vi "Lab Panel V4.82.vi"() -> ()   [LabVIEW 2013] (continued)
            n287 = local read "jig cycle"() -> (w337:dbl)
            n288 = local read "on loops"() -> (w339:dbl)
            n289 = local read "off loops"() -> (w338:dbl)
            n290 = Add(x=w324, y=w323) -> (x+y=w322:dbl)
            n291 = Add(x=w339, y=w338) -> (x+y=w325:dbl)
            n292 = Greater Or Equal?(x=w337, y=w325) -> (x >= y?=w336:bool)
            n293 = case shown="True" w336 {
              tunnel: w335 -> [_ w372]
              tunnel: w334 -> [_ w371]
              tunnel: w333 -> [_ w370]
              tunnel: w332 -> [_ w369]
              tunnel: w331 -> [_ w368]
              tunnel: w330 -> [_ w367]
              tunnel: w329 -> [_ w366]
              tunnel: w328 -> [_ w365]
              tunnel: w327 -> [_ w364]
              tunnel: w326 -> [_ w363]
              tunnel: w322 -> [_ w362]
              frame False {
              }
              frame True {
                # "increment cycle value and convert cycles to minutes for temp rise"
                n294 = local read "JIG RELAY CYCLES"() -> (w361:T10)
                n295 = Unbundle By Name(w361) -> ("LAB01-1"=w359:dbl, "LAB01-2"=w357:dbl, "LAB02-1"=w355:dbl, "LAB02-2"=w353:dbl, "LAB03-1"=w351:dbl, "LAB03-2"=w349:dbl, "LAB04-1"=w347:dbl, "LAB04-2"=w345:dbl, "LAB05-1"=w343:dbl, "LAB05-2"=w341:dbl)
                n296 = stacked-sequence {
                  tunnel: w372 -> [w384 _ _ _ _ _ _ _ _ _]
                  tunnel: w371 -> [_ w401 _ _ _ _ _ _ _ _]
                  tunnel: w370 -> [_ _ w418 _ _ _ _ _ _ _]
                  tunnel: w369 -> [_ _ _ w435 _ _ _ _ _ _]
                  tunnel: w368 -> [_ _ _ _ w452 _ _ _ _ _]
                  tunnel: w367 -> [_ _ _ _ _ w469 _ _ _ _]
                  tunnel: w366 -> [_ _ _ _ _ _ w486 _ _ _]
                  tunnel: w365 -> [_ _ _ _ _ _ _ w503 _ _]
                  tunnel: w364 -> [_ _ _ _ _ _ _ _ w520 _]
                  tunnel: w363 -> [_ _ _ _ _ _ _ _ _ w537]
                  tunnel: w362 -> [w381 w398 w415 w432 w449 w466 w483 w500 w517 w534]
                  tunnel: w359 -> [w375 _ _ _ _ _ _ _ _ _]
                  tunnel: [w374 _ _ _ _ _ _ _ _ _] -> w358
                  tunnel: w357 -> [_ w392 _ _ _ _ _ _ _ _]
                  tunnel: [_ w391 _ _ _ _ _ _ _ _] -> w356
                  tunnel: w355 -> [_ _ w409 _ _ _ _ _ _ _]
                  tunnel: [_ _ w408 _ _ _ _ _ _ _] -> w354
                  tunnel: w353 -> [_ _ _ w426 _ _ _ _ _ _]
                  tunnel: [_ _ _ w425 _ _ _ _ _ _] -> w352
                  tunnel: w351 -> [_ _ _ _ w443 _ _ _ _ _]
                  tunnel: [_ _ _ _ w442 _ _ _ _ _] -> w350
                  tunnel: w349 -> [_ _ _ _ _ w460 _ _ _ _]
                  tunnel: [_ _ _ _ _ w459 _ _ _ _] -> w348
                  tunnel: w347 -> [_ _ _ _ _ _ w477 _ _ _]
                  tunnel: [_ _ _ _ _ _ w476 _ _ _] -> w346
                  tunnel: w345 -> [_ _ _ _ _ _ _ w494 _ _]
                  tunnel: [_ _ _ _ _ _ _ w493 _ _] -> w344
                  tunnel: w343 -> [_ _ _ _ _ _ _ _ w511 _]
                  tunnel: [_ _ _ _ _ _ _ _ w510 _] -> w342
                  tunnel: w341 -> [_ _ _ _ _ _ _ _ _ w528]
                  tunnel: [_ _ _ _ _ _ _ _ _ w527] -> w340
                  frame #0 {
                    n297 = local read "DISP LAB01-1"() -> (w379:T4)
                    n298 = Unbundle(w379) -> ("CYCLE"=w380:dbl)  [unwired: 2 out]
                    n299 = case shown="True" w384 {
                      tunnel: w380 -> [w386 w390]
                      tunnel: [w386 w389] -> w378
                      tunnel: w375 -> [w385 w388]
                      tunnel: [w385 w387] -> w374
                      frame False {
                      }
                      frame True {
                        n300 = Increment(x=w388) -> (x+1=w387:dbl)
                        n301 = Increment(x=w390) -> (x+1=w389:dbl)
                      }
                    }
                    n302 = Multiply(x=w378, y=w381) -> (x*y=w382:dbl)
                    n303 = Divide(x=w382, y=60.0) -> (x/y=w377:dbl)
                    n304 = Bundle(cluster=w379, "CYCLE"=w378, "MINS"=w377) -> (w376:T4)  [unwired: 1 in]
                    n305 = local write "DISP LAB01-1"(w376) -> ()
                  }
                  frame #1 {
                    n306 = local read "DISP LAB01-2"() -> (w396:T4)
                    n307 = Unbundle(w396) -> ("CYCLE"=w397:dbl)  [unwired: 2 out]
                    n308 = case shown="True" w401 {
                      tunnel: w397 -> [w403 w407]
                      tunnel: [w403 w406] -> w394
                      tunnel: w392 -> [w402 w405]
                      tunnel: [w402 w404] -> w391
                      frame False {
                      }
                      frame True {
                        n309 = Increment(x=w405) -> (x+1=w404:dbl)
                        n310 = Increment(x=w407) -> (x+1=w406:dbl)
                      }
                    }
                    n311 = Multiply(x=w394, y=w398) -> (x*y=w399:dbl)
                    n312 = Divide(x=w399, y=60.0) -> (x/y=w393:dbl)
                    n313 = Bundle(cluster=w396, "CYCLE"=w394, "MINS"=w393) -> (w395:T4)  [unwired: 1 in]
                    n314 = local write "DISP LAB01-2"(w395) -> ()
                  }
                  frame #2 {
                    n315 = local read "DISP LAB02-1"() -> (w413:T4)
                    n316 = Unbundle(w413) -> ("CYCLE"=w414:dbl)  [unwired: 2 out]
                    n317 = case shown="True" w418 {
                      tunnel: [w420 w424] -> w411
                      tunnel: w414 -> [w420 w423]
                      tunnel: w409 -> [w419 w422]
                      tunnel: [w419 w421] -> w408
                      frame False {
                      }
                      frame True {
                        n318 = Increment(x=w422) -> (x+1=w421:dbl)
                        n319 = Increment(x=w423) -> (x+1=w424:dbl)
                      }
                    }
                    n320 = Multiply(x=w411, y=w415) -> (x*y=w416:dbl)
                    n321 = Divide(x=w416, y=60.0) -> (x/y=w410:dbl)
                    n322 = Bundle(cluster=w413, "CYCLE"=w411, "MINS"=w410) -> (w412:T4)  [unwired: 1 in]
                    n323 = local write "DISP LAB02-1"(w412) -> ()
                  }
                  frame #3 {
                    n324 = local read "DISP LAB02-2"() -> (w430:T4)
                    n325 = Unbundle(w430) -> ("CYCLE"=w431:dbl)  [unwired: 2 out]
                    n326 = case shown="True" w435 {
                      tunnel: [w437 w441] -> w429
                      tunnel: w431 -> [w437 w440]
                      tunnel: w426 -> [w436 w439]
                      tunnel: [w436 w438] -> w425
                      frame False {
                      }
                      frame True {
                        n327 = Increment(x=w439) -> (x+1=w438:dbl)
                        n328 = Increment(x=w440) -> (x+1=w441:dbl)
                      }
                    }
                    n329 = Multiply(x=w429, y=w432) -> (x*y=w433:dbl)
                    n330 = Divide(x=w433, y=60.0) -> (x/y=w428:dbl)
                    n331 = Bundle(cluster=w430, "CYCLE"=w429, "MINS"=w428) -> (w427:T4)  [unwired: 1 in]
                    n332 = local write "DISP LAB02-2"(w427) -> ()
                  }
                  frame #4 {
                    n333 = local read "DISP LAB03-1"() -> (w447:T4)
                    n334 = Unbundle(w447) -> ("CYCLE"=w448:dbl)  [unwired: 2 out]
                    n335 = case shown="True" w452 {
                      tunnel: [w454 w458] -> w444
                      tunnel: w448 -> [w454 w457]
                      tunnel: w443 -> [w453 w456]
                      tunnel: [w453 w455] -> w442
                      frame False {
                      }
                      frame True {
                        n336 = Increment(x=w456) -> (x+1=w455:dbl)
                        n337 = Increment(x=w457) -> (x+1=w458:dbl)
                      }
                    }
                    n338 = Multiply(x=w444, y=w449) -> (x*y=w450:dbl)
                    n339 = Divide(x=w450, y=60.0) -> (x/y=w445:dbl)
                    n340 = Bundle(cluster=w447, "CYCLE"=w444, "MINS"=w445) -> (w446:T4)  [unwired: 1 in]
                    n341 = local write "DISP LAB03-1"(w446) -> ()
                  }
                  frame #5 {
                    n342 = local read "DISP LAB03-2"() -> (w464:T4)
                    n343 = Unbundle(w464) -> ("CYCLE"=w465:dbl)  [unwired: 2 out]
                    n344 = case shown="True" w469 {
                      tunnel: [w471 w475] -> w463
                      tunnel: w465 -> [w471 w474]
                      tunnel: w460 -> [w470 w473]
                      tunnel: [w470 w472] -> w459
                      frame False {
                      }
                      frame True {
                        n345 = Increment(x=w473) -> (x+1=w472:dbl)
                        n346 = Increment(x=w474) -> (x+1=w475:dbl)
                      }
                    }
                    n347 = Multiply(x=w463, y=w466) -> (x*y=w467:dbl)
                    n348 = Divide(x=w467, y=60.0) -> (x/y=w462:dbl)
                    n349 = Bundle(cluster=w464, "CYCLE"=w463, "MINS"=w462) -> (w461:T4)  [unwired: 1 in]
                    n350 = local write "DISP LAB03-2"(w461) -> ()
                  }
                  frame #6 {
                    n351 = local read "DISP LAB04-1"() -> (w481:T4)
                    n352 = Unbundle(w481) -> ("CYCLE"=w482:dbl)  [unwired: 2 out]
                    n353 = case shown="True" w486 {
                      tunnel: [w488 w492] -> w479
                      tunnel: w482 -> [w488 w491]
                      tunnel: w477 -> [w487 w490]
                      tunnel: [w487 w489] -> w476
                      frame False {
                      }
                      frame True {
                        n354 = Increment(x=w490) -> (x+1=w489:dbl)
                        n355 = Increment(x=w491) -> (x+1=w492:dbl)
                      }
                    }
                    n356 = Multiply(x=w479, y=w483) -> (x*y=w484:dbl)
                    n357 = Divide(x=w484, y=60.0) -> (x/y=w478:dbl)
                    n358 = Bundle(cluster=w481, "CYCLE"=w479, "MINS"=w478) -> (w480:T4)  [unwired: 1 in]
                    n359 = local write "DISP LAB04-1"(w480) -> ()
                  }
                  frame #7 {
                    n360 = local read "DISP LAB04-2"() -> (w498:T4)
                    n361 = Unbundle(w498) -> ("CYCLE"=w499:dbl)  [unwired: 2 out]
                    n362 = case shown="True" w503 {
                      tunnel: [w505 w509] -> w496
                      tunnel: w499 -> [w505 w508]
                      tunnel: w494 -> [w504 w507]
                      tunnel: [w504 w506] -> w493
                      frame False {
                      }
                      frame True {
                        n363 = Increment(x=w507) -> (x+1=w506:dbl)
                        n364 = Increment(x=w508) -> (x+1=w509:dbl)
                      }
                    }
                    n365 = Multiply(x=w496, y=w500) -> (x*y=w502:dbl)
                    n366 = Divide(x=w502, y=60.0) -> (x/y=w495:dbl)
                    n367 = Bundle(cluster=w498, "CYCLE"=w496, "MINS"=w495) -> (w497:T4)  [unwired: 1 in]
                    n368 = local write "DISP LAB04-2"(w497) -> ()
                  }
                  frame #8 {
                    n369 = local read "DISP LAB05-1"() -> (w515:T4)
                    n370 = Unbundle(w515) -> ("CYCLE"=w516:dbl)  [unwired: 2 out]
                    n371 = case shown="True" w520 {
                      tunnel: [w522 w526] -> w513
                      tunnel: w516 -> [w522 w525]
                      tunnel: w511 -> [w521 w524]
                      tunnel: [w521 w523] -> w510
                      frame False {
                      }
                      frame True {
                        n372 = Increment(x=w524) -> (x+1=w523:dbl)
                        n373 = Increment(x=w525) -> (x+1=w526:dbl)
                      }
                    }
                    n374 = Multiply(x=w513, y=w517) -> (x*y=w518:dbl)
                    n375 = Divide(x=w518, y=60.0) -> (x/y=w512:dbl)
                    n376 = Bundle(cluster=w515, "CYCLE"=w513, "MINS"=w512) -> (w514:T4)  [unwired: 1 in]
                    n377 = local write "DISP LAB05-1"(w514) -> ()
                  }
                  frame #9 {
                    n378 = local read "DISP LAB05-2"() -> (w533:T4)
                    n379 = Unbundle(w533) -> ("CYCLE"=w532:dbl)  [unwired: 2 out]
                    n380 = case shown="True" w537 {
                      tunnel: [w539 w543] -> w531
                      tunnel: w532 -> [w539 w542]
                      tunnel: w528 -> [w538 w541]
                      tunnel: [w538 w540] -> w527
                      frame False {
                      }
                      frame True {
                        n381 = Increment(x=w541) -> (x+1=w540:dbl)
                        n382 = Increment(x=w542) -> (x+1=w543:dbl)
                      }
                    }
                    n383 = Multiply(x=w531, y=w534) -> (x*y=w535:dbl)
                    n384 = Divide(x=w535, y=60.0) -> (x/y=w530:dbl)
                    n385 = Bundle(cluster=w533, "CYCLE"=w531, "MINS"=w530) -> (w529:T4)  [unwired: 1 in]
                    n386 = local write "DISP LAB05-2"(w529) -> ()
                  }
                }
                n387 = local write "jig cycle"(0) -> ()
                n388 = Bundle By Name(cluster=w361, "LAB01-1"=w358, "LAB01-2"=w356, "LAB02-1"=w354, "LAB02-2"=w352, "LAB03-1"=w350, "LAB03-2"=w348, "LAB04-1"=w346, "LAB04-2"=w344, "LAB05-1"=w342, "LAB05-2"=w340) -> (w360:T10)
                n389 = local write "JIG RELAY CYCLES"(w360) -> ()
              }
            }
          }
          frame #3 {
            # "START & STOP test RUN switch change, start test if true and stop test if false"
            n390 = Get Date/Time In Seconds() -> (seconds since 1Jan1904=w551:timestamp)
            n391 = local read "C drive data root dir"() -> (w544:path)
            n392 = Format Date/Time String(time format string (%c)="%b\\%a%d", seconds (now)=w551) -> (date/time string=w575:string)  [unwired: 1 in]
            n393 = Format Date/Time String(time format string (%c)="%H%M", seconds (now)=w551) -> (date/time string=w573:string)  [unwired: 1 in]
            n394 = Format Date/Time String(time format string (%c)="LabPanel%Y", seconds (now)=w551) -> (date/time string=w550:string)  [unwired: 1 in]
            n395 = Path To String(path=w544) -> (string=w547:string)
            n396 = global write "Global 1.vi" "C drive root path"(w544) -> ()
            n397 = Concatenate Strings(w547, "\\") -> (w545:string)
            n398 = event shown="[5] \"RUN LAB03-1\": Value Change" {
              selector: _ -> [_ _ _ _ _ _ _ _ _ _ _]
              dyn-events: _ -> [_ _ _ _ _ _ _ _ _ _ _]
              timeout: 10 -> [_ _ _ _ _ _ _ _ _ _ _]
              tunnel: w545 -> [_ w583 w675 w767 w859 w951 w1043 w1135 w1227 w1319 w1411]
              tunnel: w575 -> [_ w582 w674 w766 w858 w950 w1042 w1134 w1226 w1318 w1410]
              tunnel: w573 -> [_ w580 w673 w765 w857 w949 w1041 w1133 w1225 w1317 w1409]
              tunnel: w571 -> [_ w581 _ _ _ _ _ _ _ _ _]
              tunnel: w572 -> [_ _ _ _ _ _ _ _ _ _ _]
              tunnel: w570 -> [_ _ _ _ _ _ _ _ _ _ _]
              tunnel: w569 -> [_ _ w672 _ _ _ _ _ _ _ _]
              tunnel: w568 -> [_ _ _ _ _ _ _ _ _ _ _]
              tunnel: w567 -> [_ _ _ w764 _ _ _ _ _ _ _]
              tunnel: w566 -> [_ _ _ _ _ _ _ _ _ _ _]
              tunnel: w565 -> [_ _ _ _ w856 _ _ _ _ _ _]
              tunnel: w564 -> [_ _ _ _ _ _ _ _ _ _ _]
              tunnel: w563 -> [_ _ _ _ _ w948 _ _ _ _ _]
              tunnel: w562 -> [_ _ _ _ _ _ _ _ _ _ _]
              tunnel: w561 -> [_ _ _ _ _ _ w1040 _ _ _ _]
              tunnel: w560 -> [_ _ _ _ _ _ _ _ _ _ _]
              tunnel: w559 -> [_ _ _ _ _ _ _ w1132 _ _ _]
              tunnel: w558 -> [_ _ _ _ _ _ _ _ _ _ _]
              tunnel: w557 -> [_ _ _ _ _ _ _ _ w1224 _ _]
              tunnel: w556 -> [_ _ _ _ _ _ _ _ _ _ _]
              tunnel: w555 -> [_ _ _ _ _ _ _ _ _ w1316 _]
              tunnel: w554 -> [_ _ _ _ _ _ _ _ _ _ _]
              tunnel: w553 -> [_ _ _ _ _ _ _ _ _ _ w1408]
              tunnel: w550 -> [_ w579 w671 w763 w855 w947 w1039 w1131 w1223 w1315 w1407]
              tunnel: [_ w578 w670 w762 w854 w946 w1038 w1130 w1222 w1314 w1406] -> w548
              event Timeout {
                n399 = event-data() -> ()  [unwired: 1 in, 3 out]
              }
              event "RUN LAB01-1": Value Change {
                n400 = event-data() -> ("NewVal"=w577:bool)  [unwired: 1 in, 5 out]
                n401 = local write "run lab01-1"(w577) -> ()
                n402 = case shown="True" w577 {
                  tunnel: w583 -> [_ w616]
                  tunnel: w582 -> [_ w615]
                  tunnel: w581 -> [w585 w614]
                  tunnel: w580 -> [_ w613]
                  tunnel: w579 -> [_ w612]
                  tunnel: [w584 w611] -> w578
                  frame False {
                    # "stop test"
                    n403 = stacked-sequence {
                      tunnel: w585 -> [_ w597 _ _]
                      tunnel: [_ w589 _ _] -> w584
                      frame #0 {
                        n404 = local read "DISP LAB01-1"() -> (w588:T4)
                        n405 = Bundle(cluster=w588, "STATUS"="STOP") -> (w586:T4)  [unwired: 2 in]
                        n406 = local write "DISP LAB01-1"(w586) -> ()
                      }
                      frame #1 {
                        n407 = local read "DISP LAB01-1"() -> (w596:T4)
                        n408 = Unbundle(w596) -> ("CYCLE"=w594:dbl, "MINS"=w595:dbl)  [unwired: 1 out]
                        n409 = case shown="\"CYCLE TEST\"" w597 {
                          tunnel: w595 -> [_ _ w604]
                          tunnel: w594 -> [w602 w603 _]
                          tunnel: [w602 w603 w604] -> w593
                          frame "CHART TEST", Default {
                          }
                          frame "CYCLE TEST" {
                          }
                          frame "T-RISE TEST" {
                          }
                        }
                        n410 = local read "TDMS LAB01-1"() -> (w601:refnum<k34>)
                        n411 = Build Array("STOPPED") -> (w598:string[])
                        n412 = Build Array(w593) -> (w592:dbl[])
                        n413 = TDMS Write(0:w601, 5:"TEST RESULT", 7:w598, 9:w592) -> (4:w590:refnum<k34>, 15:w591:errorcluster)  [unwired: 2 in, 2 out]
                        n414 = TDMS Close(8:w591, 11:w590) -> (0:w589:errorcluster)  [unwired: 1 out]
                      }
                      frame #2 {
                        n415 = stacked-sequence {
                          tunnel: "LAB01-1" -> [w607 w609]
                          frame #0 {
                            n416 = call "sub vi - defrag tdms v1.vi"("panel id"=w607) -> ("error out"=w606:errorcluster)  [unwired: 10 in]
                            n417 = local write "data file error"(w606) -> ()
                          }
                          frame #1 {
                            n418 = call "Save data file to network drive v1.vi"("panel id"=w609) -> ("network file save error"=w608:errorcluster)  [unwired: 9 in, 1 out]
                            n419 = local write "RESULT LAB01-1"(FALSE) -> ()
                            n420 = local write "data file error"(w608) -> ()
                          }
                        }
                      }
                      frame #3 {
                      }
                    }
                  }
                  frame True {
                    # "start new test and create test file"
                    n421 = stacked-sequence {
                      seq-local: [w617 _ _ _ _] -> [_ w638 _ _ _]
                      tunnel: w616 -> [w622 _ _ _ _]
                      tunnel: w615 -> [w618 _ _ _ _]
                      tunnel: w614 -> [w632 _ _ _ _]
                      tunnel: w613 -> [w625 _ _ _ _]
                      tunnel: w612 -> [w620 _ _ _ _]
                      tunnel: [_ w639 _ _ _] -> w611
                      frame #0 {
                        w619 = "\\"
                        n422 = case shown="\"CHART TEST\", Default" w632 {
                          tunnel: ["L01-1-CHART TEST-" "L01-1-CYCLE TEST-" "L01-1-T-RISE TEST-"] -> w628
                          frame "CHART TEST", Default {
                          }
                          frame "CYCLE TEST" {
                          }
                          frame "T-RISE TEST" {
                          }
                        }
                        n423 = local read "SET LAB01-1"() -> (w627:T5)
                        n424 = Unbundle(w627) -> ("DESCRIPTION"=w626:string)  [unwired: 4 out]
                        n425 = Concatenate Strings(w622, "\\", w620, w619, w618, w619) -> (w629:string)
                        n426 = String To Path(string=w629) -> (path=w631:path)
                        n427 = Concatenate Strings(w629, w628, w626, "-", w625, ".tdms") -> (w617:string)
                        n428 = Create Folder(path (use dialog)=w631) -> (error out=w630:errorcluster)  [unwired: 2 in, 2 out]
                        n429 = call <vilib>:"Clear Errors.vi"("error in (no error)"=w630) -> ()  [unwired: 6 in, 1 out]
                        n430 = global write "Global 1.vi" "LAB01-1 FILE"(w617) -> ()
                      }
                      frame #1 {
                        n431 = String To Path(string=w638) -> (path=w636:path)
                        n432 = TDMS Open(5:FALSE, 6:FALSE, 10:T19."create or replace" ("operation (0:open)"), 11:w636) -> (0:w639:errorcluster, 3:→"TDMS LAB01-1":refnum<k34>)  [unwired: 3 in]
                      }
                      frame #2 {
                        n433 = local read "TDMS LAB01-1"() -> (w659:refnum<k34>)
                        n434 = local read "SET LAB01-1"() -> (w648:T5)
                        n435 = Build Array("Testers Name", "Description", "Set Test Cycles", "T-Rise minutes", "T-Rise Deg C") -> (w649:string[])
                        n436 = Unbundle(w648) -> ("NAME"=w647:string, "DESCRIPTION"=w646:string, "CYCLES"=w645:dbl, "T-RISE mins"=w644:dbl, "T-RISE deg C"=w643:dbl)
                        n437 = Number To Decimal String(number=w645) -> (decimal integer string=w658:string)  [unwired: 1 in]
                        n438 = Number To Decimal String(number=w644) -> (decimal integer string=w657:string)  [unwired: 1 in]
                        n439 = Number To Decimal String(number=w643) -> (decimal integer string=w656:string)  [unwired: 1 in]
                        n440 = Build Array(w647, w646, w658, w657, w656) -> (w655:string[])
                        n441 = TDMS Set Properties(5:w655, 7:w649, 11:w659) -> ()  [unwired: 3 in, 4 out]
                      }
                      frame #3 {
                        w660 = 0.0
                        n442 = local read "DISP LAB01-1"() -> (w663:T4)
                        n443 = Bundle(cluster=w663, "CYCLE"=w660, "MINS"=w660, "STATUS"="RUN") -> (w662:T4)
                        n444 = local write "DISP LAB01-1"(w662) -> ()
                      }
                      frame #4 {
                        n445 = local read "SIG LAB01-1"() -> (w666:T2)
                        n446 = local read "TEMP START LAB01-1"() -> (w668:cluster{"TL":dbl, "TN":dbl})
                        n447 = Unbundle(w666) -> ("Tmp Live"=w665:dbl, "Tmp Neut"=w664:dbl)  [unwired: 3 out]
                        n448 = Bundle(cluster=w668, "TL"=w665, "TN"=w664) -> (w667:cluster{"TL":dbl, "TN":dbl})
                        n449 = local write "TEMP START LAB01-1"(w667) -> ()
                      }
                    }
                  }
                }
              }
              event "RUN LAB01-2": Value Change {
                n450 = event-data() -> ("NewVal"=w669:bool)  [unwired: 1 in, 5 out]
                n451 = local write "run lab01-2"(w669) -> ()
                n452 = case shown="True" w669 {
                  tunnel: w675 -> [_ w708]
                  tunnel: w674 -> [_ w707]
                  tunnel: w672 -> [w677 w706]
                  tunnel: w673 -> [_ w705]
                  tunnel: w671 -> [_ w704]
                  tunnel: [w676 w703] -> w670
                  frame False {
                    # "stop test"
                    n453 = stacked-sequence {
                      tunnel: w677 -> [w686 _]
                      tunnel: [w678 _] -> w676
                      frame #0 {
                        n454 = local read "DISP LAB01-2"() -> (w685:T4)
                        n455 = Unbundle(w685) -> ("CYCLE"=w683:dbl, "MINS"=w684:dbl)  [unwired: 1 out]
                        n456 = case shown="\"CHART TEST\", Default" w686 {
                          tunnel: w684 -> [_ _ w693]
                          tunnel: w683 -> [w691 w692 _]
                          tunnel: [w691 w692 w693] -> w682
                          frame "CHART TEST", Default {
                          }
                          frame "CYCLE TEST" {
                          }
                          frame "T-RISE TEST" {
                          }
                        }
                        n457 = local read "TDMS LAB01-2"() -> (w690:refnum<k34>)
                        n458 = Build Array("STOPPED") -> (w687:string[])
                        n459 = Build Array(w682) -> (w681:dbl[])
                        n460 = TDMS Write(0:w690, 5:"TEST RESULT", 7:w687, 9:w681) -> (4:w679:refnum<k34>, 15:w680:errorcluster)  [unwired: 2 in, 2 out]
                        n461 = TDMS Close(8:w680, 11:w679) -> (0:w678:errorcluster)  [unwired: 1 out]
                      }
                      frame #1 {
                        n462 = local read "DISP LAB01-2"() -> (w697:T4)
                        n463 = stacked-sequence {
                          tunnel: "LAB01-2" -> [w699 w701]
                          frame #0 {
                            n464 = call "sub vi - defrag tdms v1.vi"("panel id"=w699) -> ("error out"=w698:errorcluster)  [unwired: 10 in]
                            n465 = local write "data file error"(w698) -> ()
                          }
                          frame #1 {
                            n466 = call "Save data file to network drive v1.vi"("panel id"=w701) -> ("network file save error"=w700:errorcluster)  [unwired: 9 in, 1 out]
                            n467 = local write "RESULT LAB01-2"(FALSE) -> ()
                            n468 = local write "data file error"(w700) -> ()
                          }
                        }
                        n469 = Bundle(cluster=w697, "STATUS"="STOP") -> (w695:T4)  [unwired: 2 in]
                        n470 = local write "DISP LAB01-2"(w695) -> ()
                      }
                    }
                  }
                  frame True {
                    # "start new test and create test file"
                    n471 = stacked-sequence {
                      seq-local: [w709 _ _ _ _] -> [_ w734 _ _ _]
                      tunnel: w708 -> [w714 _ _ _ _]
                      tunnel: w707 -> [w711 _ _ _ _]
                      tunnel: w706 -> [w724 _ _ _ _]
                      tunnel: w705 -> [w717 _ _ _ _]
                      tunnel: w704 -> [w712 _ _ _ _]
                      tunnel: [_ w728 _ _ _] -> w703
                      frame #0 {
                        w710 = "\\"
                        n472 = local read "SET LAB01-2"() -> (w719:T5)
                        n473 = case shown="\"CYCLE TEST\"" w724 {
                          tunnel: ["L01-2-CHART TEST-" "L01-2-CYCLE TEST-" "L01-2-T-RISE TEST-"] -> w720
                          frame "CHART TEST", Default {
                          }
                          frame "CYCLE TEST" {
                          }
                          frame "T-RISE TEST" {
                          }
                        }
                        n474 = Unbundle(w719) -> ("DESCRIPTION"=w718:string)  [unwired: 4 out]
                        n475 = Concatenate Strings(w714, "\\", w712, w710, w711, w710) -> (w721:string)
                        n476 = String To Path(string=w721) -> (path=w723:path)
                        n477 = Concatenate Strings(w721, w720, w718, "-", w717, ".tdms") -> (w709:string)
                        n478 = Create Folder(path (use dialog)=w723) -> (error out=w722:errorcluster)  [unwired: 2 in, 2 out]
                        n479 = global write "Global 1.vi" "LAB01-2 FILE"(w709) -> ()
                        n480 = call <vilib>:"Clear Errors.vi"("error in (no error)"=w722) -> ()  [unwired: 6 in, 1 out]
                      }
                      frame #1 {
                        n481 = String To Path(string=w734) -> (path=w729:path)
                        n482 = TDMS Open(5:FALSE, 6:FALSE, 10:T19."create or replace" ("operation (0:open)"), 11:w729) -> (0:w728:errorcluster, 3:→"TDMS LAB01-2":refnum<k34>)  [unwired: 3 in]
                      }
                      frame #2 {
                        n483 = local read "SET LAB01-2"() -> (w740:T5)
                        n484 = local read "TDMS LAB01-2"() -> (w751:refnum<k34>)
                        n485 = Build Array("Testers Name", "Description", "Set Test Cycles", "T-Rise minutes", "T-Rise Deg C") -> (w741:string[])
                        n486 = Unbundle(w740) -> ("NAME"=w739:string, "DESCRIPTION"=w738:string, "CYCLES"=w737:dbl, "T-RISE mins"=w736:dbl, "T-RISE deg C"=w735:dbl)
                        n487 = Number To Decimal String(number=w737) -> (decimal integer string=w750:string)  [unwired: 1 in]
                        n488 = Number To Decimal String(number=w736) -> (decimal integer string=w749:string)  [unwired: 1 in]
                        n489 = Number To Decimal String(number=w735) -> (decimal integer string=w748:string)  [unwired: 1 in]
                        n490 = Build Array(w739, w738, w750, w749, w748) -> (w747:string[])
                        n491 = TDMS Set Properties(5:w747, 7:w741, 11:w751) -> ()  [unwired: 3 in, 4 out]
                      }
                      frame #3 {
                        w753 = 0.0
                        n492 = local read "DISP LAB01-2"() -> (w755:T4)
                        n493 = Bundle(cluster=w755, "CYCLE"=w753, "MINS"=w753, "STATUS"="RUN") -> (w754:T4)
                        n494 = local write "DISP LAB01-2"(w754) -> ()
                      }
                      frame #4 {
                        n495 = local read "SIG LAB01-2"() -> (w758:T2)
                        n496 = local read "TEMP START LAB01-2"() -> (w760:cluster{"TL":dbl, "TN":dbl})
                        n497 = Unbundle(w758) -> ("Tmp Live"=w757:dbl, "Tmp Neut"=w756:dbl)  [unwired: 3 out]
                        n498 = Bundle(cluster=w760, "TL"=w757, "TN"=w756) -> (w759:cluster{"TL":dbl, "TN":dbl})
                        n499 = local write "TEMP START LAB01-2"(w759) -> ()
                      }
                    }
                  }
                }
              }
              event "RUN LAB02-1": Value Change {
                n500 = event-data() -> ("NewVal"=w761:bool)  [unwired: 1 in, 5 out]
                n501 = local write "run lab02-1"(w761) -> ()
                n502 = case shown="True" w761 {
                  tunnel: w767 -> [_ w800]
                  tunnel: w766 -> [_ w799]
                  tunnel: w764 -> [w769 w798]
                  tunnel: w765 -> [_ w797]
                  tunnel: w763 -> [_ w796]
                  tunnel: [w768 w795] -> w762
                  frame False {
                    # "stop test"
                    n503 = stacked-sequence {
                      tunnel: w769 -> [w778 _]
                      tunnel: [w770 _] -> w768
                      frame #0 {
                        n504 = local read "DISP LAB02-1"() -> (w777:T4)
                        n505 = Unbundle(w777) -> ("CYCLE"=w775:dbl, "MINS"=w776:dbl)  [unwired: 1 out]
                        n506 = case shown="\"CYCLE TEST\"" w778 {
                          tunnel: w776 -> [_ _ w785]
                          tunnel: w775 -> [w783 w784 _]
                          tunnel: [w783 w784 w785] -> w774
                          frame "CHART TEST", Default {
                          }
                          frame "CYCLE TEST" {
                          }
                          frame "T-RISE TEST" {
                          }
                        }
                        n507 = local read "TDMS LAB02-1"() -> (w782:refnum<k34>)
                        n508 = Build Array("STOPPED") -> (w779:string[])
                        n509 = Build Array(w774) -> (w773:dbl[])
                        n510 = TDMS Write(0:w782, 5:"TEST RESULT", 7:w779, 9:w773) -> (4:w771:refnum<k34>, 15:w772:errorcluster)  [unwired: 2 in, 2 out]
                        n511 = TDMS Close(8:w772, 11:w771) -> (0:w770:errorcluster)  [unwired: 1 out]
                      }
                      frame #1 {
                        n512 = local read "DISP LAB02-1"() -> (w789:T4)
                        n513 = stacked-sequence {
                          tunnel: "LAB02-1" -> [w791 w793]
                          frame #0 {
                            n514 = call "sub vi - defrag tdms v1.vi"("panel id"=w791) -> ("error out"=w790:errorcluster)  [unwired: 10 in]
                            n515 = local write "data file error"(w790) -> ()
                          }
                          frame #1 {
                            n516 = local write "RESULT LAB02-1"(FALSE) -> ()
                            n517 = call "Save data file to network drive v1.vi"("panel id"=w793) -> ("network file save error"=w792:errorcluster)  [unwired: 9 in, 1 out]
                            n518 = local write "data file error"(w792) -> ()
                          }
                        }
                        n519 = Bundle(cluster=w789, "STATUS"="STOP") -> (w787:T4)  [unwired: 2 in]
                        n520 = local write "DISP LAB02-1"(w787) -> ()
                      }
                    }
                  }
                  frame True {
                    # "start new test and create test file"
                    n521 = stacked-sequence {
                      seq-local: [w801 _ _ _ _] -> [_ w826 _ _ _]
                      tunnel: w800 -> [w806 _ _ _ _]
                      tunnel: w799 -> [w803 _ _ _ _]
                      tunnel: w798 -> [w816 _ _ _ _]
                      tunnel: w797 -> [w809 _ _ _ _]
                      tunnel: w796 -> [w804 _ _ _ _]
                      tunnel: [_ w820 _ _ _] -> w795
                      frame #0 {
                        w802 = "\\"
                        n522 = local read "SET LAB02-1"() -> (w811:T5)
                        n523 = case shown="\"CYCLE TEST\"" w816 {
                          tunnel: ["L02-1-CHART TEST-" "L02-1-CYCLE TEST-" "L02-1-T-RISE TEST-"] -> w812
                          frame "CHART TEST", Default {
                          }
                          frame "CYCLE TEST" {
                          }
                          frame "T-RISE TEST" {
                          }
                        }
                        n524 = Unbundle(w811) -> ("DESCRIPTION"=w810:string)  [unwired: 4 out]
                        n525 = Concatenate Strings(w806, "\\", w804, w802, w803, w802) -> (w813:string)
                        n526 = String To Path(string=w813) -> (path=w815:path)
                        n527 = Concatenate Strings(w813, w812, w810, "-", w809, ".tdms") -> (w801:string)
                        n528 = Create Folder(path (use dialog)=w815) -> (error out=w814:errorcluster)  [unwired: 2 in, 2 out]
                        n529 = global write "Global 1.vi" "LAB02-1 FILE"(w801) -> ()
                        n530 = call <vilib>:"Clear Errors.vi"("error in (no error)"=w814) -> ()  [unwired: 6 in, 1 out]
                      }
                      frame #1 {
                        n531 = String To Path(string=w826) -> (path=w821:path)
                        n532 = TDMS Open(5:FALSE, 6:FALSE, 10:T19."create or replace" ("operation (0:open)"), 11:w821) -> (0:w820:errorcluster, 3:→"TDMS LAB02-1":refnum<k34>)  [unwired: 3 in]
                      }
                      frame #2 {
                        n533 = local read "SET LAB02-1"() -> (w832:T5)
                        n534 = local read "TDMS LAB02-1"() -> (w843:refnum<k34>)
                        n535 = Build Array("Testers Name", "Description", "Set Test Cycles", "T-Rise minutes", "T-Rise Deg C") -> (w833:string[])
                        n536 = Unbundle(w832) -> ("NAME"=w831:string, "DESCRIPTION"=w830:string, "CYCLES"=w829:dbl, "T-RISE mins"=w828:dbl, "T-RISE deg C"=w827:dbl)
                        n537 = Number To Decimal String(number=w829) -> (decimal integer string=w842:string)  [unwired: 1 in]
                        n538 = Number To Decimal String(number=w828) -> (decimal integer string=w841:string)  [unwired: 1 in]
                        n539 = Number To Decimal String(number=w827) -> (decimal integer string=w840:string)  [unwired: 1 in]
                        n540 = Build Array(w831, w830, w842, w841, w840) -> (w839:string[])
                        n541 = TDMS Set Properties(5:w839, 7:w833, 11:w843) -> ()  [unwired: 3 in, 4 out]
                      }
                      frame #3 {
                        w845 = 0.0
                        n542 = local read "DISP LAB02-1"() -> (w847:T4)
                        n543 = Bundle(cluster=w847, "CYCLE"=w845, "MINS"=w845, "STATUS"="RUN") -> (w846:T4)
                        n544 = local write "DISP LAB02-1"(w846) -> ()
                      }
                      frame #4 {
                        n545 = local read "SIG LAB02-1"() -> (w850:T2)
                        n546 = local read "TEMP START LAB02-1"() -> (w852:cluster{"TL":dbl, "TN":dbl})
                        n547 = Unbundle(w850) -> ("Tmp Live"=w849:dbl, "Tmp Neut"=w848:dbl)  [unwired: 3 out]
                        n548 = Bundle(cluster=w852, "TL"=w849, "TN"=w848) -> (w851:cluster{"TL":dbl, "TN":dbl})
                        n549 = local write "TEMP START LAB02-1"(w851) -> ()
                      }
                    }
                  }
                }
              }
              event "RUN LAB02-2": Value Change {
                n550 = event-data() -> ("NewVal"=w853:bool)  [unwired: 1 in, 5 out]
                n551 = local write "run lab02-2"(w853) -> ()
                n552 = case shown="True" w853 {
                  tunnel: w859 -> [_ w892]
                  tunnel: w858 -> [_ w891]
                  tunnel: w856 -> [w861 w890]
                  tunnel: w857 -> [_ w889]
                  tunnel: w855 -> [_ w888]
                  tunnel: [w860 w887] -> w854
                  frame False {
                    # "stop test"
                    n553 = stacked-sequence {
                      tunnel: w861 -> [w870 _]
                      tunnel: [w862 _] -> w860
                      frame #0 {
                        n554 = local read "DISP LAB02-2"() -> (w869:T4)
                        n555 = Unbundle(w869) -> ("CYCLE"=w867:dbl, "MINS"=w868:dbl)  [unwired: 1 out]
                        n556 = case shown="\"CYCLE TEST\"" w870 {
                          tunnel: w868 -> [_ _ w877]
                          tunnel: w867 -> [w875 w876 _]
                          tunnel: [w875 w876 w877] -> w866
                          frame "CHART TEST", Default {
                          }
                          frame "CYCLE TEST" {
                          }
                          frame "T-RISE TEST" {
                          }
                        }
                        n557 = local read "TDMS LAB02-2"() -> (w874:refnum<k34>)
                        n558 = Build Array("STOPPED") -> (w871:string[])
                        n559 = Build Array(w866) -> (w865:dbl[])
                        n560 = TDMS Write(0:w874, 5:"TEST RESULT", 7:w871, 9:w865) -> (4:w863:refnum<k34>, 15:w864:errorcluster)  [unwired: 2 in, 2 out]
                        n561 = TDMS Close(8:w864, 11:w863) -> (0:w862:errorcluster)  [unwired: 1 out]
                      }
                      frame #1 {
                        n562 = local read "DISP LAB02-2"() -> (w881:T4)
                        n563 = stacked-sequence {
                          tunnel: "LAB02-2" -> [w883 w885]
                          frame #0 {
                            n564 = call "sub vi - defrag tdms v1.vi"("panel id"=w883) -> ("error out"=w882:errorcluster)  [unwired: 10 in]
                            n565 = local write "data file error"(w882) -> ()
                          }
                          frame #1 {
                            n566 = call "Save data file to network drive v1.vi"("panel id"=w885) -> ("network file save error"=w884:errorcluster)  [unwired: 9 in, 1 out]
                            n567 = local write "RESULT LAB02-2"(FALSE) -> ()
                            n568 = local write "data file error"(w884) -> ()
                          }
                        }
                        n569 = Bundle(cluster=w881, "STATUS"="STOP") -> (w879:T4)  [unwired: 2 in]
                        n570 = local write "DISP LAB02-2"(w879) -> ()
                      }
                    }
                  }
                  frame True {
                    # "start new test and create test file"
                    n571 = stacked-sequence {
                      seq-local: [w893 _ _ _ _] -> [_ w918 _ _ _]
                      tunnel: w892 -> [w898 _ _ _ _]
                      tunnel: w891 -> [w895 _ _ _ _]
                      tunnel: w890 -> [w908 _ _ _ _]
                      tunnel: w889 -> [w901 _ _ _ _]
                      tunnel: w888 -> [w896 _ _ _ _]
                      tunnel: [_ w912 _ _ _] -> w887
                      frame #0 {
                        w894 = "\\"
                        n572 = local read "SET LAB02-2"() -> (w903:T5)
                        n573 = case shown="\"CYCLE TEST\"" w908 {
                          tunnel: ["L02-2-CHART TEST-" "L02-2-CYCLE TEST-" "L02-2-T-RISE TEST-"] -> w904
                          frame "CHART TEST", Default {
                          }
                          frame "CYCLE TEST" {
                          }
                          frame "T-RISE TEST" {
                          }
                        }
                        n574 = Unbundle(w903) -> ("DESCRIPTION"=w902:string)  [unwired: 4 out]
                        n575 = Concatenate Strings(w898, "\\", w896, w894, w895, w894) -> (w905:string)
                        n576 = String To Path(string=w905) -> (path=w907:path)
                        n577 = Concatenate Strings(w905, w904, w902, "-", w901, ".tdms") -> (w893:string)
                        n578 = Create Folder(path (use dialog)=w907) -> (error out=w906:errorcluster)  [unwired: 2 in, 2 out]
                        n579 = global write "Global 1.vi" "LAB02-2 FILE"(w893) -> ()
                        n580 = call <vilib>:"Clear Errors.vi"("error in (no error)"=w906) -> ()  [unwired: 6 in, 1 out]
                      }
                      frame #1 {
                        n581 = String To Path(string=w918) -> (path=w913:path)
                        n582 = TDMS Open(5:FALSE, 6:FALSE, 10:T19."create or replace" ("operation (0:open)"), 11:w913) -> (0:w912:errorcluster, 3:→"TDMS LAB02-2":refnum<k34>)  [unwired: 3 in]
                      }
                      frame #2 {
                        n583 = local read "SET LAB02-2"() -> (w924:T5)
                        n584 = local read "TDMS LAB02-2"() -> (w935:refnum<k34>)
                        n585 = Build Array("Testers Name", "Description", "Set Test Cycles", "T-Rise minutes", "T-Rise Deg C") -> (w925:string[])
                        n586 = Unbundle(w924) -> ("NAME"=w923:string, "DESCRIPTION"=w922:string, "CYCLES"=w921:dbl, "T-RISE mins"=w920:dbl, "T-RISE deg C"=w919:dbl)
                        n587 = Number To Decimal String(number=w921) -> (decimal integer string=w934:string)  [unwired: 1 in]
                        n588 = Number To Decimal String(number=w920) -> (decimal integer string=w933:string)  [unwired: 1 in]
                        n589 = Number To Decimal String(number=w919) -> (decimal integer string=w932:string)  [unwired: 1 in]
                        n590 = Build Array(w923, w922, w934, w933, w932) -> (w931:string[])
                        n591 = TDMS Set Properties(5:w931, 7:w925, 11:w935) -> ()  [unwired: 3 in, 4 out]
                      }
                      frame #3 {
                        w937 = 0.0
                        n592 = local read "DISP LAB02-2"() -> (w939:T4)
                        n593 = Bundle(cluster=w939, "CYCLE"=w937, "MINS"=w937, "STATUS"="RUN") -> (w938:T4)
                        n594 = local write "DISP LAB02-2"(w938) -> ()
                      }
                      frame #4 {
                        n595 = local read "SIG LAB02-2"() -> (w942:T2)
                        n596 = local read "TEMP START LAB02-2"() -> (w944:cluster{"TL":dbl, "TN":dbl})
                        n597 = Unbundle(w942) -> ("Tmp Live"=w941:dbl, "Tmp Neut"=w940:dbl)  [unwired: 3 out]
                        n598 = Bundle(cluster=w944, "TL"=w941, "TN"=w940) -> (w943:cluster{"TL":dbl, "TN":dbl})
                        n599 = local write "TEMP START LAB02-2"(w943) -> ()
                      }
                    }
                  }
                }
              }
              event "RUN LAB03-1": Value Change {
                n600 = event-data() -> ("NewVal"=w945:bool)  [unwired: 1 in, 5 out]
                n601 = local write "run lab03-1"(w945) -> ()
                n602 = case shown="True" w945 {
                  tunnel: w951 -> [_ w984]
                  tunnel: w950 -> [_ w983]
                  tunnel: w948 -> [w953 w982]
                  tunnel: w949 -> [_ w981]
                  tunnel: w947 -> [_ w980]
                  tunnel: [w952 w979] -> w946
                  frame False {
                    # "stop test"
                    n603 = stacked-sequence {
                      tunnel: w953 -> [w962 _]
                      tunnel: [w954 _] -> w952
                      frame #0 {
                        n604 = local read "DISP LAB03-1"() -> (w961:T4)
                        n605 = Unbundle(w961) -> ("CYCLE"=w959:dbl, "MINS"=w960:dbl)  [unwired: 1 out]
                        n606 = case shown="\"CYCLE TEST\"" w962 {
                          tunnel: w960 -> [_ _ w969]
                          tunnel: w959 -> [w967 w968 _]
                          tunnel: [w967 w968 w969] -> w958
                          frame "CHART TEST", Default {
                          }
                          frame "CYCLE TEST" {
                          }
                          frame "T-RISE TEST" {
                          }
                        }
                        n607 = local read "TDMS LAB03-1"() -> (w966:refnum<k34>)
                        n608 = Build Array("STOPPED") -> (w963:string[])
                        n609 = Build Array(w958) -> (w957:dbl[])
                        n610 = TDMS Write(0:w966, 5:"TEST RESULT", 7:w963, 9:w957) -> (4:w955:refnum<k34>, 15:w956:errorcluster)  [unwired: 2 in, 2 out]
                        n611 = TDMS Close(8:w956, 11:w955) -> (0:w954:errorcluster)  [unwired: 1 out]
                      }
                      frame #1 {
                        n612 = local read "DISP LAB03-1"() -> (w973:T4)
                        n613 = stacked-sequence {
                          tunnel: "LAB03-1" -> [w975 w977]
                          frame #0 {
                            n614 = call "sub vi - defrag tdms v1.vi"("panel id"=w975) -> ("error out"=w974:errorcluster)  [unwired: 10 in]
                            n615 = local write "data file error"(w974) -> ()
                          }
                          frame #1 {
                            n616 = call "Save data file to network drive v1.vi"("panel id"=w977) -> ("network file save error"=w976:errorcluster)  [unwired: 9 in, 1 out]
                            n617 = local write "RESULT LAB03-1"(FALSE) -> ()
                            n618 = local write "data file error"(w976) -> ()
                          }
                        }
                        n619 = Bundle(cluster=w973, "STATUS"="STOP") -> (w971:T4)  [unwired: 2 in]
                        n620 = local write "DISP LAB03-1"(w971) -> ()
                      }
                    }
                  }
                  frame True {
                    # "start new test and create test file"
                    n621 = stacked-sequence {
                      seq-local: [w985 _ _ _ _] -> [_ w1010 _ _ _]
                      tunnel: w984 -> [w990 _ _ _ _]
                      tunnel: w983 -> [w987 _ _ _ _]
                      tunnel: w982 -> [w1000 _ _ _ _]
                      tunnel: w981 -> [w993 _ _ _ _]
                      tunnel: w980 -> [w988 _ _ _ _]
                      tunnel: [_ w1004 _ _ _] -> w979
                      frame #0 {
                        w986 = "\\"
                        n622 = local read "SET LAB03-1"() -> (w995:T5)
                        n623 = case shown="\"T-RISE TEST\"" w1000 {
                          tunnel: ["L03-1-CHART TEST-" "L03-1-CYCLE TEST-" "L03-1-T-RISE TEST-"] -> w996
                          frame "CHART TEST", Default {
                          }
                          frame "CYCLE TEST" {
                          }
                          frame "T-RISE TEST" {
                          }
                        }
                        n624 = Unbundle(w995) -> ("DESCRIPTION"=w994:string)  [unwired: 4 out]
                        n625 = Concatenate Strings(w990, "\\", w988, w986, w987, w986) -> (w997:string)
                        n626 = String To Path(string=w997) -> (path=w999:path)
                        n627 = Concatenate Strings(w997, w996, w994, "-", w993, ".tdms") -> (w985:string)
